vi "test_Add Array Existing Ch. Name.vi"(8 "error in (no error)":errorcluster, 11 "TestCase in":refnum<class "Instrument Addon Scripting API Channels Unit Tests.lvclass">) -> (0 "error out":errorcluster, 3 "TestCase out":refnum<class "Instrument Addon Scripting API Channels Unit Tests.lvclass">)   [LabVIEW 2018, in "Instrument Addon Scripting API Channels Unit Tests.lvclass"]
uses:
  Instrument Addon Scripting API Channels Unit Tests.lvclass
  APIs/Scripting API/TypeDefs/Array Enumerated List Settings.ctl
  APIs/Scripting API/TypeDefs/Array Element.ctl
  Instrument Addon Scripting API Channels Unit Tests.lvclass/Instrument Addon Scripting API Channels Unit Tests.ctl
  Addon/Addon Shared/SubVIs/Constants.vi
  <vilib>/NI/NI VeriStand Advanced SysDef API/_SubVIs/SysDef.Search.GUID.vi
  <vilib>/NI/NI VeriStand Advanced SysDef API/_SubVIs/SysDef.Search.GUIDs.vi
  APIs/Scripting API/Channels/Create Data Channel - Array - Enumerated List.vi
  <vilib>/addons/_JKI Toolkits/VI Tester/TestCase.llb/TestCase.lvclass
  Instrument Addon Scripting API Test Assets/Instrument Addon Scripting API Test Assets.lvclass
  <vilib>/NI/NI VeriStand Advanced SysDef API/SysDef API/Advanced System Definition.lvlib
  Addon/Addon Shared/Instrument Addon Shared.lvlib
  APIs/Scripting API/Instrument Addon Scripting API.lvlib
  C:/Program Files (x86)/National Instruments/LabVIEW 2018/vi.lib/addons/_JKI Toolkits/VI Tester/TestCase.llb/TestCase.lvclass
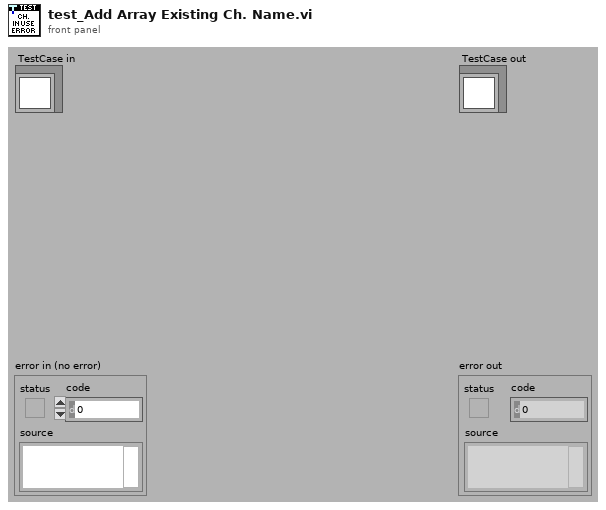
[diagram p1: front panel]
types:
  T1 = typedef "Instrument Addon Scripting API.lvlib/Array Enumerated List Settings.ctl" = cluster{"Elements":T2[], "Enumerated List":string[], "Delimiter":string}
  T2 = typedef "Instrument Addon Scripting API.lvlib/Array Element.ctl" = cluster{"Name":string, "Default Value":dbl, "Units":string}
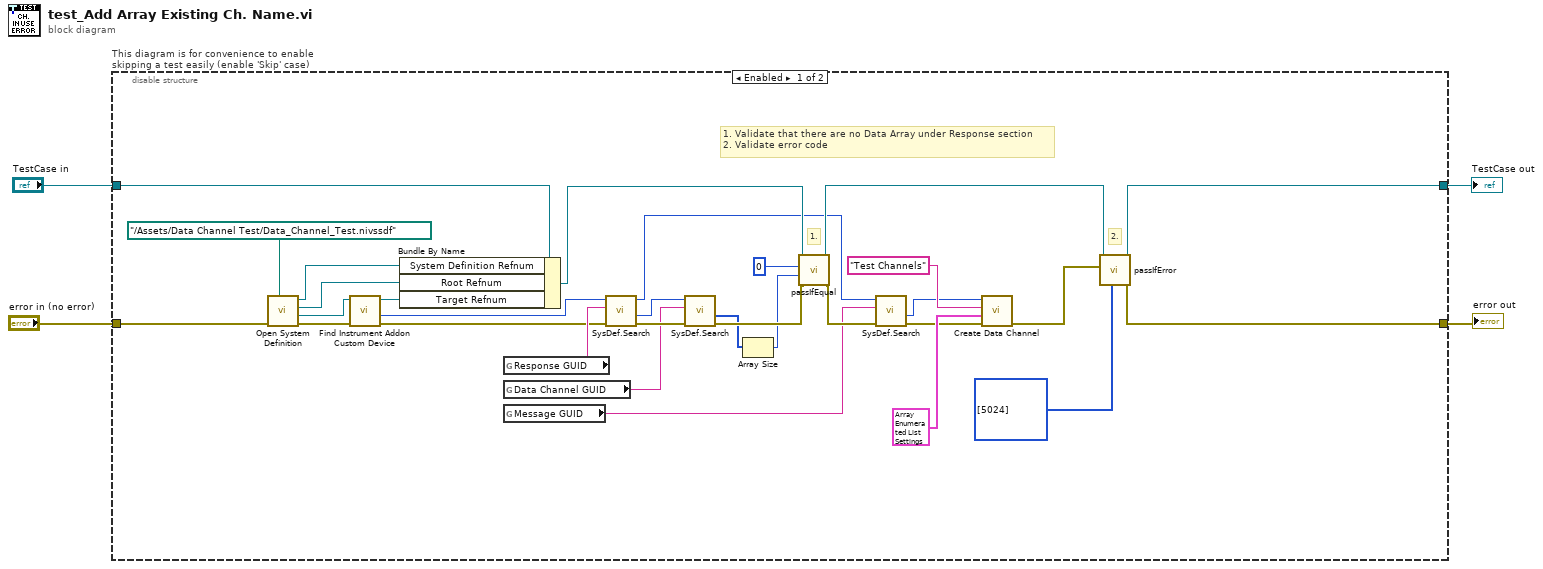
[diagram p0: block diagram]
diagram:
  n1 = disable-structure "This diagram is for convenience to enable skipping a test easily (enable 'Skip' case)" shown="Enabled" {
    disable-tunnel: "TestCase in" -> [w15 w39]
    disable-tunnel: [w17 w37] -> w1
    disable-tunnel: [w18 w38] -> w3
    disable-tunnel: "error in (no error)" -> [w32 w36]
    frame Enabled {
      # "2."
      # "1. Validate that there are no Data Array under Response section\n2. Validate error code"
      # "1."
      n2 = call "Open System Definition.vi"("error in (no error)"=w32, "System Definition File"=path "../Assets/Data Channel Test/Data_Channel_Test.nivssdf") -> ("error out"=w35:errorcluster, "Target Refnum"=w34:refnum<k24>, "Root Refnum"=w13:refnum<k24>, "System Definition Refnum"=w14:refnum<k24>)  [unwired: 6 in]
      n3 = call "Find Instrument Addon Custom Device.vi"("error in"=w35, "target in"=w34) -> ("error out"=w10:errorcluster, "NodeID"=w31:u64, "target out"=w12:refnum<k24>)  [unwired: 7 in]
      n4 = Bundle By Name(cluster=w15, "System Definition Refnum"=w14, "Root Refnum"=w13, "Target Refnum"=w12) -> (w11:refnum<class "Instrument Addon Scripting API Channels Unit Tests.lvclass">)
      n5 = global read "Constants.vi" "Response GUID"() -> (w30:string)
      n6 = global read "Constants.vi" "Data Channel GUID"() -> (w27:string)
      n7 = global read "Constants.vi" "Message GUID"() -> (w7:string)
      n8 = call-poly <vilib>:"SysDef.Search.vi"("error in (no error)"=w10, "GUID"=w30, "nodeID"=w31) -> ("error out"=w28:errorcluster, "Value out"=w29:u64, "nodeID out"=w6:u64)  [unwired: 5 in, 1 out]
      n9 = call-poly <vilib>:"SysDef.Search.vi"("error in (no error)"=w28, "GUID"=w27, "nodeID"=w29) -> ("error out"=w25:errorcluster, "Values Out"=w24:u64[])  [unwired: 5 in, 2 out]
      n10 = Array Size(array=w24) -> (size(s)=w23:i32)
      n11 = call-dynamic "passIfEqual.vi"("error in (no error)"=w25, "y"=w23, "x"=0 ("size(s)"), "TestCase in"=w11) -> ("error out"=w9:errorcluster, "TestCase out"=w26:refnum<class "Instrument Addon Scripting API Channels Unit Tests.lvclass">)  [unwired: 6 in]
      n12 = call-poly <vilib>:"SysDef.Search.vi"("error in (no error)"=w9, "GUID"=w7, "nodeID"=w6) -> ("error out"=w8:errorcluster, "Value out"=w5:u64)  [unwired: 5 in, 2 out]
      n13 = call-poly "Create Data Channel.vi"("Error In"=w8, "Settings"=T1 {"Elements"=[{"Name"="Scale", "Default Value"=10.0, "Units"="ms"}, {"Name"="Scale", "Default Value"=15.0, "Units"="ms"}], "Enumerated List"=["EnumListElement"], "Delimiter"="-"}, "Name"="Test Channels", "Message Refnum In"=w5) -> ("Error Out"=w16:errorcluster)  [unwired: 5 in, 2 out]
      n14 = call-dynamic "passIfError.vi"("passing error codes (default = any error code)"=i32[] [5024], "error"=w16, "TestCase in"=w26) -> ("error out"=w18:errorcluster, "TestCase out"=w17:refnum<class "Instrument Addon Scripting API Channels Unit Tests.lvclass">)  [unwired: 7 in]
    }
    frame Disabled {
      # "skip test result while test is under development"
      n15 = call <vilib>:"skip.vi"("error in (no error)"=w36, "TestCase in"=w39) -> ("error out"=w38:errorcluster, "TestCase out"=w37:refnum<class "Instrument Addon Scripting API Channels Unit Tests.lvclass">)  [unwired: 8 in]
    }
  }
  "error out" <- w3
  "TestCase out" <- w1
